vi "Global_CMD_ACT_Data In.vi"() -> ()   [LabVIEW 2023, in "2024 Elevator_ACT.lvlib"]
uses:
  2024 Elevator_ACT.lvlib
  Cluster_CMD_ACT_Data.ctl
panel:
  in  "CMD_ACT_Elevator_Data":T1={"Enable Compressor"=TRUE, "Elevator Down(F) Up(t)"=FALSE}
  # "The Names of the Data items in the Global Variable MUST describe who the Single Writer is\nFor Command Globals the Commander(CMD) represents Teleop or Autonomous or other command loop.\nThe naming convention for a Command Actuator Global is:   \n\nCMD_ACT_SubSystem_Data Name\n\nExample:\nCMD_ACT_Drive_Data\nCMD_ACT_Hopper_Eject Ball"
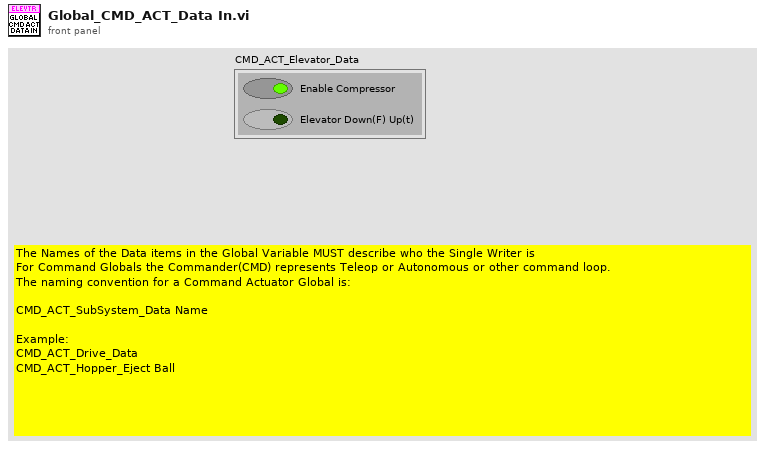
[diagram p1: front panel]
types:
  T1 = typedef "2024 Elevator_ACT.lvlib/Cluster_CMD_ACT_Data.ctl" = cluster{"Enable Compressor":bool, "Elevator Down(F) Up(t)":bool}
diagram:
